vi "New Case tester.vi"() -> ()   [LabVIEW 2020, in "Method Generation.lvlib" / "API VI Generator.lvclass"]
uses:
  API VI Generator.lvclass
  API VI Generator.lvclass/API VI Generator.ctl
panel:
  in  "error in (no error)":errorcluster
  out "error out":errorcluster
  out "output cluster":refnum<class "API VI Generator.lvclass">
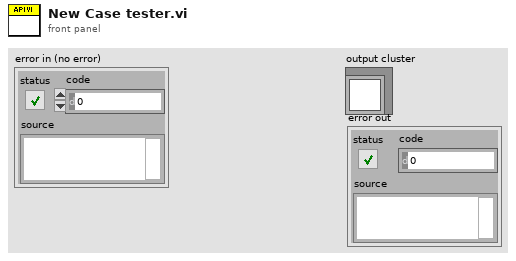
[diagram p1: front panel]
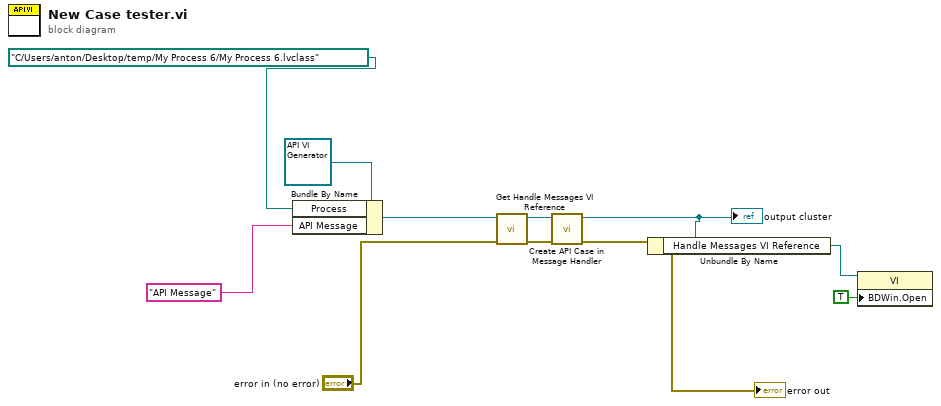
[diagram p0: block diagram]
diagram:
  n1 = Bundle By Name(cluster=refnum<class "API VI Generator.lvclass"> refnum ("New Getter Dialog In"), "Process"=path "C:/Users/anton/Desktop/temp/My Process 6/My Process 6.lvclass" ("class path"), "API Message"="API Message" ("Attribute Name")) -> (w2:refnum<class "API VI Generator.lvclass">)
  n2 = call "Get Handle Messages VI Reference.vi"("error in (no error)"="error in (no error)", "Setter Generator In"=w2) -> ("error out"=w6:errorcluster, "Setter Generator Out"=w8:refnum<class "API VI Generator.lvclass">)  [unwired: 8 in]
  n3 = call "Create API Case in Message Handler.vi"("error in (no error)"=w6, "Setter Generator In"=w8) -> ("error out"=→"error out":errorcluster, "Setter Generator Out"=w5:refnum<class "API VI Generator.lvclass">)  [unwired: 8 in]
  "output cluster" <- w5
  n4 = Unbundle By Name(w5) -> ("Handle Messages VI Reference"=w4:refnum<vi>)
  n5 = property class="VI"(reference=w4, "BDWin.Open"=TRUE ("Block Diagram Window:Open")) -> ()  [unwired: 1 in, 2 out]
